vi "Tool Data.ObjectsUpdated.vi"(8 "error in (no error)":errorcluster, 10 "Objects Updated":T1, 11 "Tool Data":refnum<class "Tool Data.lvclass">) -> (0 "error out":errorcluster, 3 "Tool Data out":refnum<class "Tool Data.lvclass">)   [LabVIEW 2019, in "Tool Data.lvclass"]
doc: "---------------------------------------------------------------\nJKI State Machine Objects™\nhttp://jki.net/state-machine-objects/\nCopyright (C) 2005-2015, JKI <info@jki.net>\nALL RIGHTS RESERVEDJKI State Machine Objects (SMO) 1.0.0.4\nJKI - JKI\nCopyright (c) 2015, JKI"
uses:
  Tool Data.lvclass
  Typedefs/PublicEvents--Tool Data.Objects Updated.ctl
  Tool Path/Tool Path.lvclass
  Tool Funnel/Tool Funnel.lvclass
  Tool Rectangle/Tool Rectangle.lvclass
  Tool Dot/Tool Dots.lvclass
  Tool Data.lvclass/Tool Data.ctl
panel:
  # "For instructions on how to use the JKI State Machine Objects, examples and video tutorials, visit:\nhttp://jki.net/state-machine-objects/\n\nJKI State Machine Objects™\nhttp://jki.net/state-machine-objects/\nCopyright (C) 2005-2015, JKI <info@jki.net>\nALL RIGHTS RESERVED"
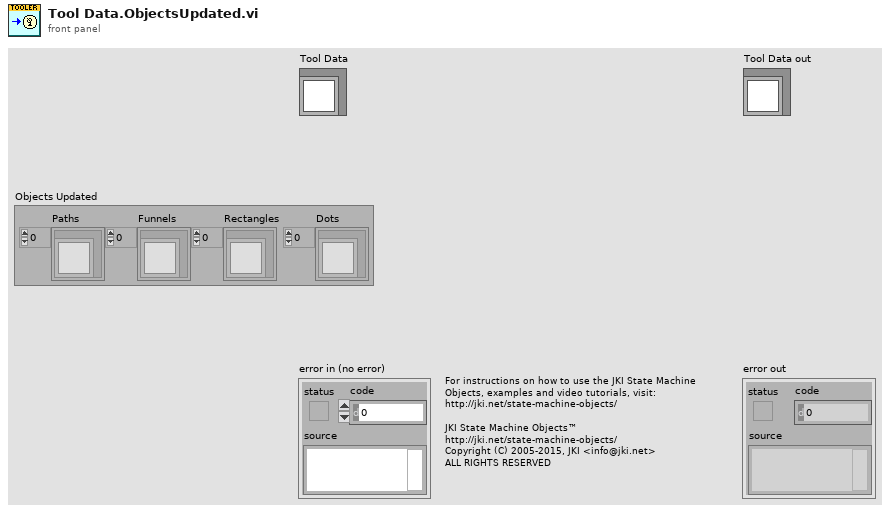
[diagram p1: front panel]
types:
  T1 = typedef "Tool Data.lvclass/PublicEvents--Tool Data.Objects Updated.ctl" = cluster{"Paths":refnum<class "Tool Path.lvclass">[], "Funnels":refnum<class "Tool Funnel.lvclass">[], "Rectangles":refnum<class "Tool Rectangle.lvclass">[], "Dots":refnum<class "Tool Dots.lvclass">[]}
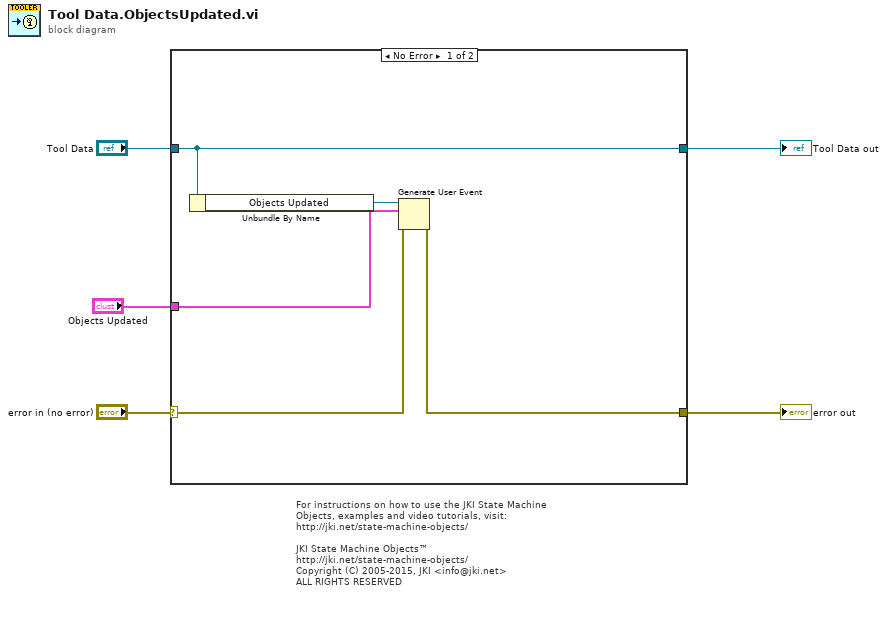
[diagram p0: block diagram]
diagram:
  # "For instructions on how to use the JKI State Machine Objects, examples and video tutorials, visit:\nhttp://jki.net/state-machine-objects/\n\nJKI State Machine Objects™\nhttp://jki.net/state-machine-objects/\nCopyright (C) 2005-2015, JKI <info@jki.net>\nALL RIGHTS RESERVED"
  n1 = case shown="No Error" "error in (no error)" {
    selector: "error in (no error)" -> [w10 w12]
    tunnel: [w7 w12] -> w4
    tunnel: [w6 w11] -> w5
    tunnel: "Tool Data" -> [w6 w11]
    tunnel: "Objects Updated" -> [w9 _]
    frame No Error {
      n2 = Unbundle By Name(w6) -> ("Objects Updated"=w8:refnum<user-event>)
      n3 = Generate User Event(user event=w8, event data cluster=w9, error in=w10) -> (error out=w7:errorcluster)  [unwired: 1 in, 1 out]
    }
    frame Error {
    }
  }
  "error out" <- w4
  "Tool Data out" <- w5
